vi "Get Info Analog In Trigger.vi"(8 "error in (no error)":errorcluster, 11 "hdwf":i32) -> (0 "error out":errorcluster, 2 "pfstrigsrc":i32, 3 "hdwf out":i32)   [LabVIEW 2012, in "AnalogDiscSDKLv.lvlib"]
doc: "extern \"C\" __declspec(dllexport) int GetInfo_AnalogIn_Trigger(HDWF hdwf, int* pfstrigsrc);"
uses:
  <instrlib>/AnalogDiscSDKLv/AnalogDiscSDKLv.lvlib
  <instrlib>/AnalogDiscSDKLv/AnalogDiscSDKLv.dll
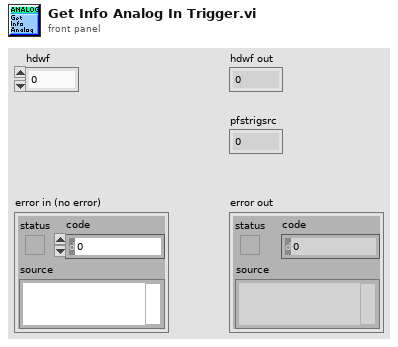
[diagram p1: front panel]
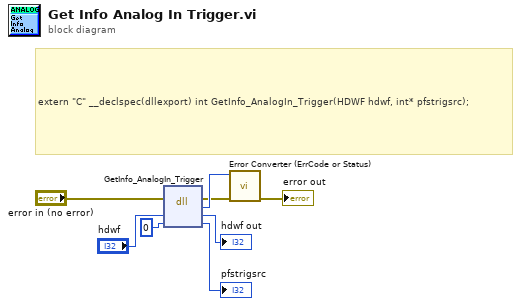
[diagram p0: block diagram]
diagram:
  # "extern \"C\" __declspec(dllexport) int GetInfo_AnalogIn_Trigger(HDWF hdwf, int* pfstrigsrc);"
  n1 = dll-call lib="C:/Program Files (x86)/National Instruments/LabVIEW 2012/instr.lib/AnalogDiscSDKLv/AnalogDiscSDKLv.*" fn="GetInfo_AnalogIn_Trigger"(error in="error in (no error)", "hdwf"="hdwf", "pfstrigsrc"=0) -> (error out=w2:errorcluster, w3:i32, "hdwf"=→"hdwf out":i32, "pfstrigsrc"=→"pfstrigsrc":i32)  [unwired: 2 in, 1 out]
  n2 = call <instrlib>:"Error Converter (ErrCode or Status).vi"("error in (no error)"=w2, "error code"=w3) -> ("error out"=→"error out":errorcluster)  [unwired: 9 in]
